vi "Log Error.vi"(8 "error in (no error)":errorcluster, 9 "Level":string, 10 "Description":string, 11 "Car Wash Controller in":refnum<class "Car Wash Controller.lvclass">) -> (0 "error out":errorcluster, 3 "Car Wash Controller out":refnum<class "Car Wash Controller.lvclass">)   [LabVIEW 2012, in "Car Wash Controller.lvlib" / "Car Wash Controller.lvclass"]
uses:
  Car Wash Controller.lvclass
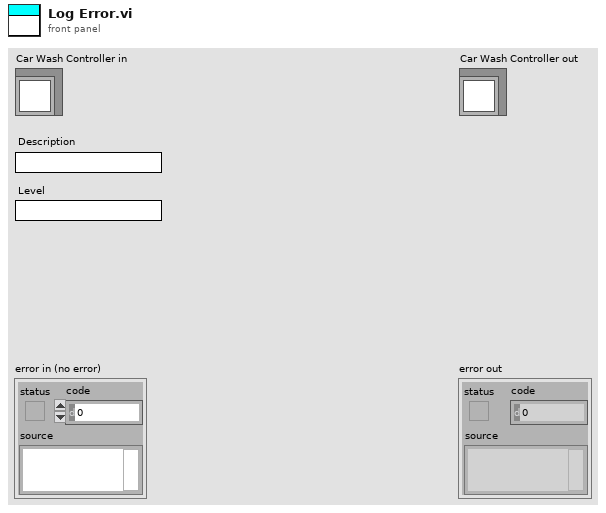
[diagram p1: front panel]
types:
  T1 = typedef "Car Wash Controller.lvlib/Car Wash Controller.lvclass/Wash Step.ctl" = enum16{"Under Body Wash", "Bug Remover", "Pre-Soak", "High Pressure Wash", "Low Pressure Wax", "Spot Free Rince", "Tire Shine Foam", "Air Dry"}
  T2 = typedef "Car Wash Controller.lvlib/Car Wash Controller.lvclass/Vehicle Position.ctl" = enum16{"Entry", "Station 1", "Station 2", "Station 3", "Exit"}
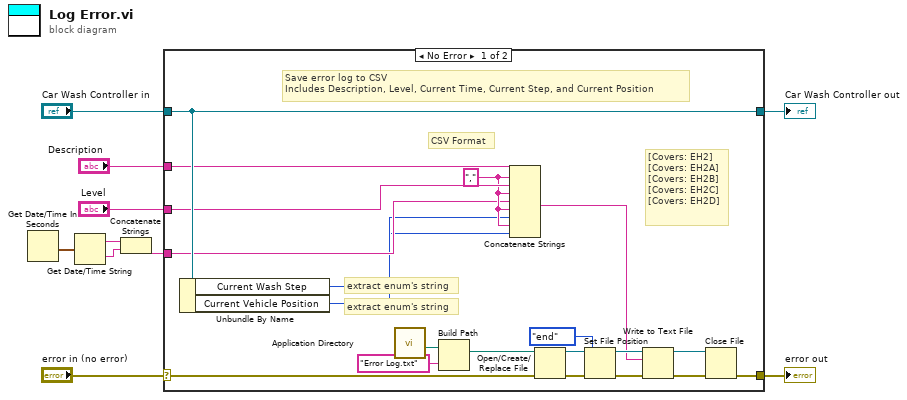
[diagram p0: block diagram]
diagram:
  n1 = Get Date/Time In Seconds() -> (seconds since 1Jan1904=w3:timestamp)
  n2 = Get Date/Time String(seconds (now)=w3) -> (date string=w5:string, time string=w4:string)  [unwired: 2 in]
  n3 = Concatenate Strings(w5, w4) -> (w1:string)
  n4 = case shown="No Error" "error in (no error)" {
    selector: "error in (no error)" -> [w18 w32]
    tunnel: [w17 w32] -> w9
    tunnel: [w30 w31] -> w7
    tunnel: "Car Wash Controller in" -> [w30 w31]
    tunnel: "Description" -> [w29 _]
    tunnel: "Level" -> [w28 _]
    tunnel: w1 -> [w26 _]
    frame No Error {
      w27 = "," ("string")
      # "[Covers: EH2]\n[Covers: EH2A]\n[Covers: EH2B]\n[Covers: EH2C]\n[Covers: EH2D]"
      # "Save error log to CSV\nIncludes Description, Level, Current Time, Current Step, and Current Position"
      # "CSV Format"
      # "extract enum's string"
      # "extract enum's string"
      n5 = Unbundle By Name(w30) -> ("Current Wash Step"=w25:T1, "Current Vehicle Position"=w24:T2)
      n6 = call <vilib>:"Application Directory.vi"() -> ("Application Directory"=w23:path)
      n7 = Build Path(base path=w23, name or relative path="Error Log.txt") -> (appended path=w16:path)
      n8 = Concatenate Strings(w29, w27, w28, w27, w26, w27, w25, w27, w24) -> (w12:string)
      n9 = Open/Create/Replace File(file path (use dialog)=w16, error in=w18) -> (refnum out=w15:refnum<file>, error out=w21:errorcluster)  [unwired: 4 in, 1 out]
      n10 = Set File Position(refnum=w15, from (0:start)=enum16{"start", "end", "current"}."end", error in=w21) -> (refnum out=w14:refnum<file>, error out=w20:errorcluster)  [unwired: 1 in]
      n11 = Write to Text File(file (use dialog)=w14, text=w12, error in=w20) -> (refnum out=w13:refnum<file>, error out=w19:errorcluster)  [unwired: 1 in, 1 out]
      n12 = Close File(refnum=w13, error in=w19) -> (error out=w17:errorcluster)  [unwired: 1 out]
    }
    frame Error {
    }
  }
  "error out" <- w9
  "Car Wash Controller out" <- w7
